vi "WRITE - File.vi"(0 "reference in":refnum<class "TDMS.lvclass">, 5 "error in (no error)":errorcluster, 7 "TDMS Path - WRITE":path) -> (14 "reference out":refnum<class "TDMS.lvclass">, 19 "error out":errorcluster)   [LabVIEW 2020, in "TDMS.lvclass"]
uses:
  TDMS.lvclass
  API/GSwFormDSP_class/functions/Attribute List.ctl
  API/GSwFormDSP_class/GSwFormDSP.lvclass
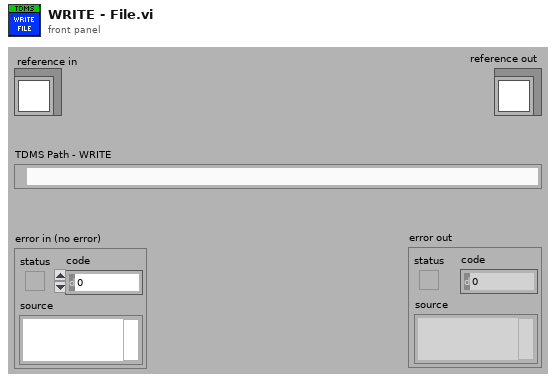
[diagram p1: front panel]
types:
  T1 = typedef "GSwFormDSP.lvclass/Attribute List.ctl" = string
  T2 = enum16{"open", "open or create", "create or replace", "create", "open (read-only)"}
  T3 = typedef "TDMS.lvclass/ObjectAttributes.ctl" = cluster{"Time Data":refnum<class "GSwFormDSP.lvclass">, "New Time Data Obj?":bool}
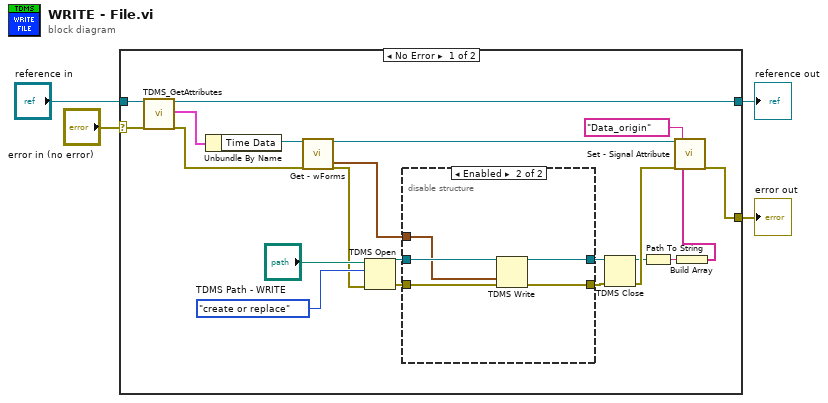
[diagram p0: block diagram]
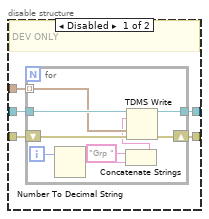
[diagram p2: hidden frame]
diagram:
  n1 = case shown="No Error" "error in (no error)" {
    selector: "error in (no error)" -> [w25 w46]
    tunnel: [w9 w46] -> w3
    tunnel: [w24 w45] -> w1
    tunnel: "reference in" -> [w22 w45]
    frame No Error {
      n2 = call "TDMS_GetAttributes.vi"("reference in"=w22, "error in (no error)"=w25) -> ("reference out"=w24:refnum<class "TDMS.lvclass">, "attributes"=w23:T3, "error out"=w20:errorcluster)  [unwired: 14 in, 1 out]
      n3 = Unbundle By Name(w23) -> ("Time Data"=w21:refnum<class "GSwFormDSP.lvclass">)
      n4 = call-dynamic "Get - wForms.vi"("reference in"=w21, "error in (no error)"=w20) -> ("wForms"=w12:waveform(dbl)[], "reference out"=w10:refnum<class "GSwFormDSP.lvclass">, "error out"=w13:errorcluster)  [unwired: 14 in, 1 out]
      n5 = TDMS Open(8:w13, 10:T2."create or replace" ("operation (0:open)"), 11:"TDMS Path - WRITE") -> (0:w16:errorcluster, 3:w17:refnum<k34>)  [unwired: 4 in]
      n6 = disable-structure shown="Enabled" {
        disable-tunnel: [w30 w43] -> w19
        disable-tunnel: [w29 w44] -> w18
        disable-tunnel: w17 -> [w28 w41]
        disable-tunnel: w16 -> [w27 w42]
        disable-tunnel: w12 -> [w26 w40]
        frame Disabled {
          # "DEV ONLY"
          n7 = for {
            tunnel: [w38] -> w29
            tunnel: w28 -> [w37]
            tunnel: w26 -> [w35] mode=indexing
            shift-right: [w39] -> w30
            shift-left: w27 -> [w36]
            i -> [w34]
            n8 = Number To Decimal String(number=w34) -> (decimal integer string=w33:string)  [unwired: 1 in]
            n9 = Concatenate Strings("Grp " ("string"), w33) -> (w31:string)
            n10 = TDMS Write(0:w37, 5:w31, 9:w35, 11:w36) -> (4:w38:refnum<k34>, 15:w39:errorcluster)  [unwired: 2 in, 2 out]
          }
        }
        frame Enabled {
          n11 = TDMS Write(0:w41, 9:w40, 11:w42) -> (4:w44:refnum<k34>, 15:w43:errorcluster)  [unwired: 3 in, 2 out]
        }
      }
      n12 = TDMS Close(8:w19, 11:w18) -> (0:w11:errorcluster, 3:w8:path)
      n13 = Path To String(path=w8) -> (string=w7:string)
      n14 = Build Array(w7) -> (w6:string[])
      n15 = call-dynamic "Set - Signal Attribute.vi"("reference in"=w10, "error in (no error)"=w11, "wForm Attributes"=T1 "Data_origin", "Attribute"=w6) -> ("error out"=w9:errorcluster)  [unwired: 14 in, 1 out]
    }
    frame Error {
    }
  }
  "error out" <- w3
  "reference out" <- w1
